vi "Base64_Decode.vi"(10 "error in (no error)":errorcluster, 11 "Base64 String":string) -> (2 "error out":errorcluster, 3 "Decoded String":string)   [LabVIEW 2013, in "Serializer.Base64.lvclass"]
uses:
  Serializer.Base64.lvclass
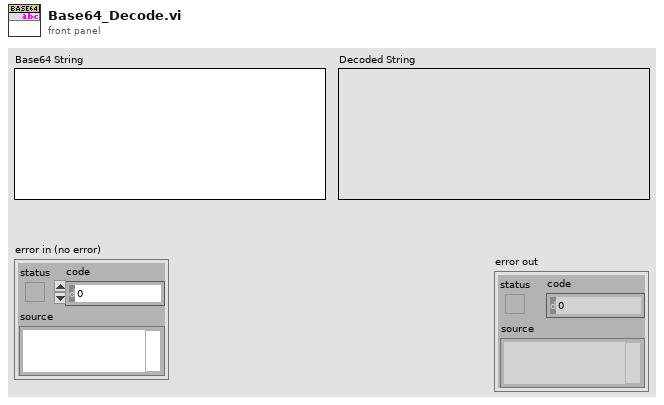
[diagram p1: front panel]
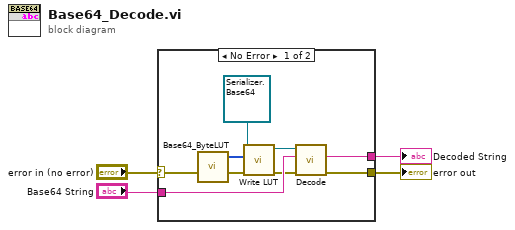
[diagram p0: block diagram]
diagram:
  n1 = case shown="No Error" "error in (no error)" {
    selector: "error in (no error)" -> [w10 w13]
    tunnel: [w5 _] -> w2
    tunnel: "Base64 String" -> [w8 _]
    tunnel: [w6 w13] -> w1
    frame No Error {
      n2 = call "Base64_ByteLUT.vi"() -> ("U8 LUT"=w12:u32[])  [unwired: 11 in]
      n3 = call "Write LUT.vi"("error in (no error)"=w10, "LUT"=w12, "Serializer.Base64 in"=refnum<class "Serializer.Base64.lvclass"> refnum ("Serializer.Base64.lvclass")) -> ("error out"=w7:errorcluster, "Serializer.Base64 out"=w9:refnum<class "Serializer.Base64.lvclass">)  [unwired: 7 in]
      n4 = call "Decode.vi"("error in (no error)"=w7, "Base64 String"=w8, "Serializer.Base64 in"=w9) -> ("error out"=w6:errorcluster, "decoded string"=w5:string)  [unwired: 6 in, 1 out]
    }
    frame Error {
    }
  }
  "Decoded String" <- w2
  "error out" <- w1
